vi "Alt_Alpha_Ver 2.0.vi"() -> ()   [LabVIEW 2015]
uses:
  <instrlib>/Keithley 622x LV 2009/Configure/Units/Typedefs/KE622x -- Voltage Meas Units.ctl
  <instrlib>/Keithley 622x LV 2009/Configure/2182 -A/Low Level/Typedefs/KE2182 -- Voltage Ranges.ctl
  <instrlib>/Keithley 622x LV 2009/Configure/2182 -A/Low Level/Typedefs/KE2182 -- Filter Type.ctl
  <instrlib>/Keithley 622x LV 2009/Configure/2182 -A/Low Level/Typedefs/KE2182 -- Filter Count.ctl
  <instrlib>/Keithley 622x LV 2009/Configure/2182 -A/Low Level/Typedefs/KE2182 -- Filter Window.ctl
  <instrlib>/Keithley 622x LV 2009/Configure/2182 -A/Low Level/Typedefs/KE2182 -- NPLCs.ctl
  <instrlib>/Keithley 622x LV 2009/Configure/Units/Typedefs/KE6221 -- PDelta Power Meas Type.ctl
  <instrlib>/Keithley 622x LV 2009/Configure/Delta PDelta DCon Modes/Typedefs/KE6221 -- PDelta Mode Params.ctl
  <instrlib>/Keithley 622x LV 2009/Configure/Delta PDelta DCon Modes/Low Level/Typedefs/KE622x -- Delta PDelta Mode High Level.ctl
  <instrlib>/Keithley 622x LV 2009/Configure/Delta PDelta DCon Modes/Low Level/Typedefs/KE622x -- Delta PDelta Mode Low Level.ctl
  <instrlib>/Keithley 622x LV 2009/Configure/Delta PDelta DCon Modes/Low Level/Typedefs/KE6221 -- PDelta Mode Pulse Width.ctl
  <instrlib>/Keithley 622x LV 2009/Configure/Delta PDelta DCon Modes/Low Level/Typedefs/KE6221 -- PDelta Mode Source Delay.ctl
  <instrlib>/Keithley 622x LV 2009/Configure/Delta PDelta DCon Modes/Low Level/Typedefs/KE622x -- Delta PDelta Mode Num Cycles Mode.ctl
  <instrlib>/Keithley 622x LV 2009/Configure/Delta PDelta DCon Modes/Low Level/Typedefs/KE622x -- Delta PDelta Mode Num Cycles.ctl
  <instrlib>/Keithley 622x LV 2009/Configure/Delta PDelta DCon Modes/Low Level/Typedefs/KE6221 -- PDelta Mode Ranging Mode.ctl
  <instrlib>/Keithley 622x LV 2009/Configure/Delta PDelta DCon Modes/Low Level/Typedefs/KE6221 -- PDelta Mode Num Low Meas.ctl
  <instrlib>/Keithley 622x LV 2009/Configure/Delta PDelta DCon Modes/Low Level/Typedefs/KE6221 -- PDelta Mode Pulse Period.ctl
  <instrlib>/Keithley 622x LV 2009/Configure/Format/Typedefs/KE622x -- Optional Meas Elements.ctl
  <instrlib>/Keithley 622x LV 2009/Configure/Trace Buf/Low Level/Typedefs/KE622x -- Trace Buf.ctl
  <instrlib>/Keithley 622x LV 2009/Configure/Delta PDelta DCon Modes/Typedefs/KE622x -- Delta Mode Params.ctl
  <instrlib>/Keithley 622x LV 2009/Configure/Delta PDelta DCon Modes/Low Level/Typedefs/KE622x -- Delta DCon Mode Delay.ctl
  <instrlib>/Keithley 622x LV 2009/Utility/Typedefs/KE622x -- Instrument Type.ctl
  <instrlib>/Keithley 622x LV 2009/Keithley 622x.lvlib
panel:
  out "FILE":refnum<file>
  out "Reading":sgl[](array[numeric])
  out "Trace Buf":T1 {"Average Voltage (V)" format="%.3p"; "Source Val (A)" format="%.3p"; "Timestamp (secs)" format="%.3f"; "Reading" format="%.7f"}
  in  "Meas Elements To Return":T2={"Timstamp?"=TRUE, "Reading Num?"=TRUE, "Source Value?"=FALSE, "Compliance?"=FALSE, "Average Voltage?"=FALSE}
  in  "stop":bool
  in  "Check For SCPI Errors? (T)":bool=TRUE
  in  "Power Meas Type":T3
  in  "2812 -A Params In":T9={"Auto Range?"=FALSE, "Man / Selected\nRange"=enum."10mV", "Enable Digital\nFilter?"=FALSE, "Filter Type"=enum."Moving", "Filter Count"=10, "Filter\nWindow (%)"=0.01, "Enable Analog\nFilter?"=FALSE, "NPLCs"=5} {"Filter\nWindow (%)" min=0.0 max=10.0 step=0.01 format="%.2f"; "Filter Count" min=1 max=100; "NPLCs" min=1 max=10}
  in  "Measurement Units":T10
  in  "Measurements control":enum32{"PULSE", " DELTA"}(tab)
  in  "Pulsed Delta Mode Params In":T11={"High Level (A)"=0.001, "Low Level (A)"=0.0, "Pulse Width (s)"=0.00011, "Source Delay (s)"=1.6e-05, "Num Cycles Mode"=enum."Infinite", "Finite Count"=1, "Ranging Mode"=enum."Best", "Num Low Meas Per Cycle"=enum."1", "Pulse Period (Num PLCs)"=5, "Pulse Sweep Mode Enabled?"=FALSE} {"Pulse Period (Num PLCs)" min=5 max=999990; "Source Delay (s)" min=1.6e-05 max=0.011966 format="%.3p"; "Pulse Width (s)" min=5e-05 max=0.012 format="%.3p"; "Finite Count" min=2 max=65536; "Low Level (A)" min=-0.105 max=0.0 format="%.3p"; "High Level (A)" min=0.0 max=0.105 format="%.3p"}
  in  "Delta Mode Params In":T21={"High Level (A)"=0.001, "Low Level (A)"=-0.001, "Delay (s)"=0.002, "Num Cycles Mode"=enum."Finite Count", "Finite Count"=1, "Abort On\nCompliance?"=FALSE, "Cold Swithing\nMode Enabled?"=FALSE} {"Finite Count" min=1 max=65536; "Low Level (A)" min=-0.105 max=0.0 format="%.3p"; "High Level (A)" min=0.0 max=0.105 format="%.3p"; "Delay (s)" min=0.001 max=9999.999 format="%.3f"}
  in  "Comments":string
  in  "Folder \nPrename":string
  # "Keithley  6221 & 2182A Measurement System"
  # "FILE CONFIGURATION"
  # "PRE EXPERIMENT CONFIGS"
  # "*** NOTE:  \"Average Voltage\"\nis only available for Differential\nConductance measurements."
  # "*** NOTE:  \"Average Voltage\"\nis only available for Differential\nConductance measurements."
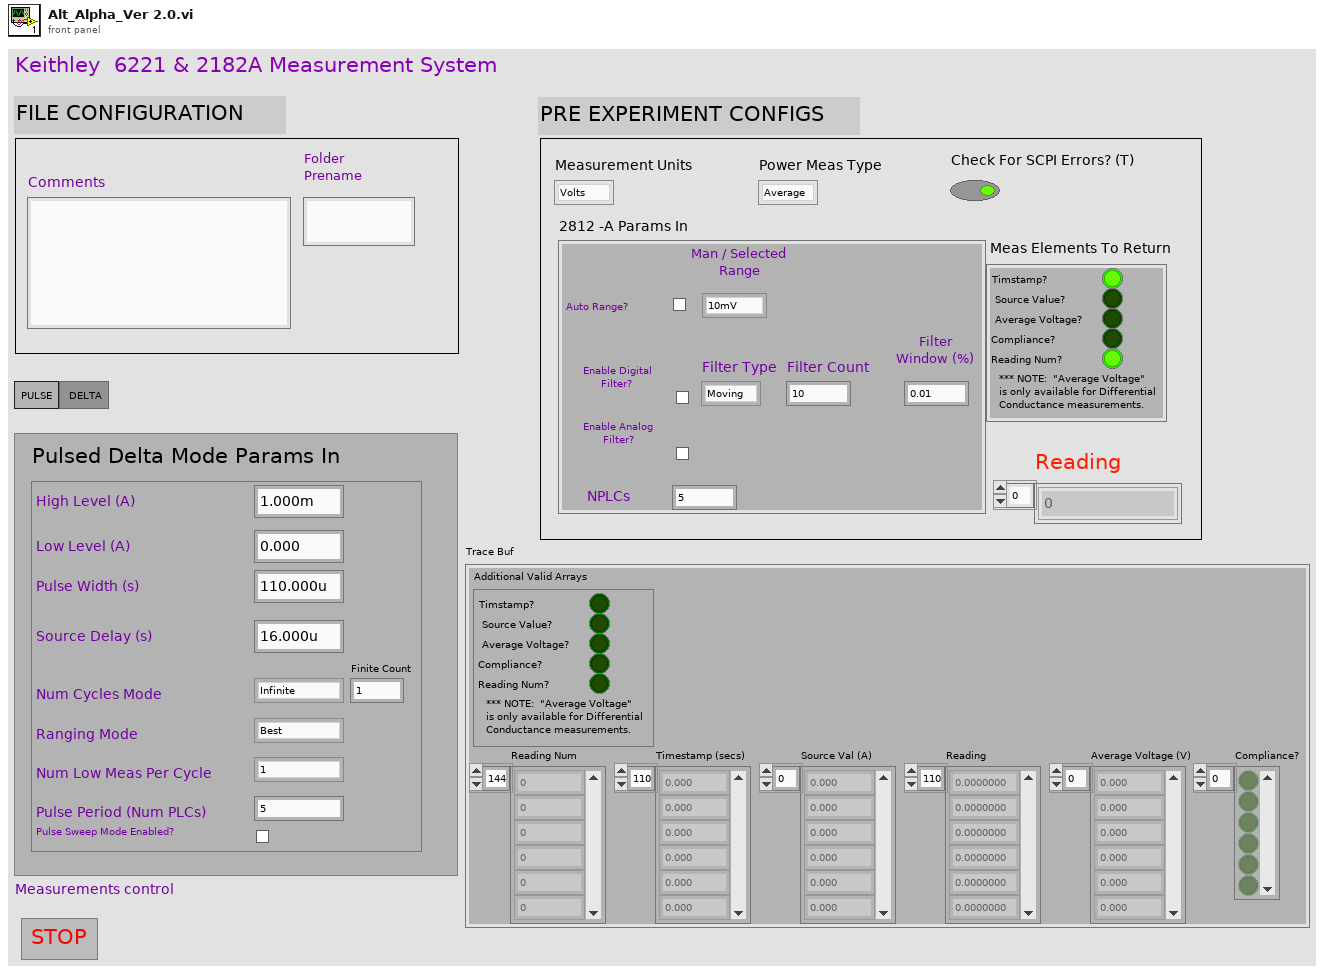
[diagram p1: front panel]
types:
  T1 = typedef "Keithley 622x.lvlib/KE622x -- Trace Buf.ctl" = cluster{"Additional Valid Arrays":T2, "Reading Num":u32[], "Timestamp (secs)":sgl[], "Source Val (A)":sgl[], "Reading":sgl[], "Average Voltage (V)":sgl[], "Compliance?":bool[]}
  T2 = typedef "Keithley 622x.lvlib/KE622x -- Optional Meas Elements.ctl" = cluster{"Timstamp?":bool, "Reading Num?":bool, "Source Value?":bool, "Compliance?":bool, "Average Voltage?":bool}
  T3 = typedef "Keithley 622x.lvlib/KE6221 -- PDelta Power Meas Type.ctl" = enum16{"Average", "Peak"}
  T4 = typedef "Keithley 622x.lvlib/KE2182 -- Voltage Ranges.ctl" = enum16{"10mV", "100mV", "1V", "10V", "100V"}
  T5 = typedef "Keithley 622x.lvlib/KE2182 -- Filter Type.ctl" = enum16{"Moving", "Repeat"}
  T6 = typedef "Keithley 622x.lvlib/KE2182 -- Filter Count.ctl" = u32
  T7 = typedef "Keithley 622x.lvlib/KE2182 -- Filter Window.ctl" = dbl
  T8 = typedef "Keithley 622x.lvlib/KE2182 -- NPLCs.ctl" = u32
  T9 = cluster{"Auto Range?":bool, "Man / Selected\nRange":T4, "Enable Digital\nFilter?":bool, "Filter Type":T5, "Filter Count":T6, "Filter\nWindow (%)":T7, "Enable Analog\nFilter?":bool, "NPLCs":T8}
  T10 = typedef "Keithley 622x.lvlib/KE622x -- Voltage Meas Units.ctl" = enum16{"Volts", "Ohms", "Watts", "Siemens"}
  T11 = typedef "Keithley 622x.lvlib/KE6221 -- PDelta Mode Params.ctl" = cluster{"High Level (A)":T12, "Low Level (A)":T13, "Pulse Width (s)":T14, "Source Delay (s)":T15, "Num Cycles Mode":T16, "Finite Count":T17, "Ranging Mode":T18, "Num Low Meas Per Cycle":T19, "Pulse Period (Num PLCs)":T20, "Pulse Sweep Mode Enabled?":bool}
  T12 = typedef "Keithley 622x.lvlib/KE622x -- Delta PDelta Mode High Level.ctl" = dbl
  T13 = typedef "Keithley 622x.lvlib/KE622x -- Delta PDelta Mode Low Level.ctl" = dbl
  T14 = typedef "Keithley 622x.lvlib/KE6221 -- PDelta Mode Pulse Width.ctl" = dbl
  T15 = typedef "Keithley 622x.lvlib/KE6221 -- PDelta Mode Source Delay.ctl" = dbl
  T16 = typedef "Keithley 622x.lvlib/KE622x -- Delta PDelta Mode Num Cycles Mode.ctl" = enum16{"Finite Count", "Infinite"}
  T17 = typedef "Keithley 622x.lvlib/KE622x -- Delta PDelta Mode Num Cycles.ctl" = u32
  T18 = typedef "Keithley 622x.lvlib/KE6221 -- PDelta Mode Ranging Mode.ctl" = enum16{"Best", "Fixed"}
  T19 = typedef "Keithley 622x.lvlib/KE6221 -- PDelta Mode Num Low Meas.ctl" = enum16{"1", "2"}
  T20 = typedef "Keithley 622x.lvlib/KE6221 -- PDelta Mode Pulse Period.ctl" = u32
  T21 = typedef "Keithley 622x.lvlib/KE622x -- Delta Mode Params.ctl" = cluster{"High Level (A)":T12, "Low Level (A)":T13, "Delay (s)":T22, "Num Cycles Mode":T16, "Finite Count":T17, "Abort On\nCompliance?":bool, "Cold Swithing\nMode Enabled?":bool}
  T22 = typedef "Keithley 622x.lvlib/KE622x -- Delta DCon Mode Delay.ctl" = dbl
  T23 = typedef "Keithley 622x.lvlib/KE622x -- Instrument Type.ctl" = enum16{"KE6220", "KE6221"}
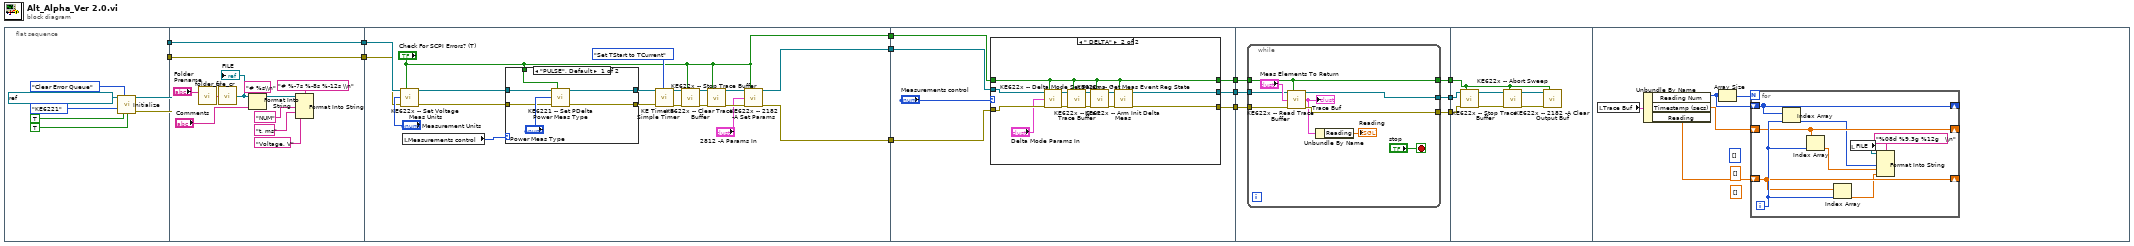
[diagram p0: block diagram]
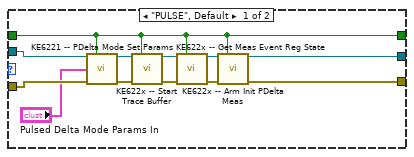
[diagram p3: hidden frame]
diagram:
  n1 = flat-sequence {
    tunnel: [w15] -> w4
    tunnel: [w14] -> w2
    tunnel: w4 -> [w32]
    tunnel: [w32] -> w3
    tunnel: w2 -> [w31]
    tunnel: [w31] -> w1
    tunnel: w3 -> [w50]
    tunnel: w1 -> [w49]
    tunnel: [w40] -> w13
    tunnel: [w39] -> w12
    tunnel: ["Check For SCPI Errors? (T)"] -> w11
    tunnel: w13 -> [w64]
    tunnel: w12 -> [w65]
    tunnel: w11 -> [w63]
    tunnel: [w62] -> w10
    tunnel: [w61] -> w9
    tunnel: [w60] -> w8
    tunnel: w10 -> [w96]
    tunnel: w9 -> [w95]
    tunnel: w8 -> [w94]
    tunnel: [w93] -> w7
    tunnel: [w92] -> w6
    tunnel: [w91] -> w5
    tunnel: w7 -> [w108]
    tunnel: w6 -> [w107]
    tunnel: w5 -> [w106]
    frame #0 {
      n2 = call <instrlib>:"Initialize.vi"("VISA resource name"=refnum<visa-resource-name> "DC_AC_Current_Source_6221", "Error Queue Option"=enum16{"Clear Error Queue", "Error Query"}."Clear Error Queue", "Instrument Type"=KE622x_--_Instrument_Type."KE6221", "ID Query? (T)"=TRUE, "Reset? (T)"=TRUE) -> ("VISA resource name out"=w15:refnum<visa-resource-name>, "error out"=w14:errorcluster)  [unwired: 9 in]
    }
    frame #1 {
      n3 = call "folder_cr.vi"("Name"="Folder \nPrename") -> ("String"=w23:string)
      n4 = call "file_cr.vi"("String"=w23) -> ("refnum out"=w21:refnum<file>)
      "FILE" <- w21
      n5 = Format Into String(format string="# %s\\n", initial string=w21, "Comments") -> (resulting string=w28:refnum<file>)  [unwired: 1 in, 1 out]
      n6 = Format Into String(format string="# %-7s %-8s %-12s \\n", initial string=w28, "NUM" ("input 1"), "t, ms" ("input 2"), "Voltage, V" ("input 3")) -> ()  [unwired: 1 in, 2 out]
    }
    frame #2 {
      n7 = call <instrlib>:"KE622x -- Set Voltage Meas Units.vi"("Resource In"=w50, "Check For SCPI Errors? (T)"="Check For SCPI Errors? (T)", "Voltage Meas Units"="Measurement Units", "error in (no error)"=w49) -> ("Resource Out (dupl)"=w36:refnum<visa-resource-name>, "error out"=w35:errorcluster)  [unwired: 10 in]
      n8 = local read "Measurements control"() -> (w38:enum32{"PULSE", " DELTA"})
      n9 = case shown="\"PULSE\", Default" w38 {
        tunnel: "Check For SCPI Errors? (T)" -> [w56 _]
        tunnel: w36 -> [w55 w59]
        tunnel: w35 -> [w54 w58]
        tunnel: [w53 w59] -> w34
        tunnel: [w52 w58] -> w33
        frame "PULSE", Default {
          n10 = call <instrlib>:"KE6221 -- Set PDelta Power Meas Type.vi"("6221 Resource In"=w55, "Check For SCPI Errors? (T)"=w56, "Power Meas Type"="Power Meas Type", "error in (no error)"=w54) -> ("6221 Resource Out (dupl)"=w53:refnum<visa-resource-name>, "error out"=w52:errorcluster)  [unwired: 10 in]
        }
        frame " DELTA" {
        }
      }
      n11 = call <instrlib>:"KE Timer -- Simple Timer.vi"("Resource In"=w34, "error in (no error)"=w33, "Action"=enum16{"Set TStart to TCurrent", "Get Deltas"}."Set TStart to TCurrent") -> ("Resource Out (dupl)"=w47:refnum<visa-resource-name>, "error out (dupl)"=w46:errorcluster)  [unwired: 7 in, 8 out]
      n12 = call <instrlib>:"KE622x -- Stop Trace Buffer.vi"("Resource In"=w47, "Check For SCPI Errors? (T)"="Check For SCPI Errors? (T)", "error in (no error)"=w46) -> ("Resource Out (dupl)"=w45:refnum<visa-resource-name>, "error out"=w44:errorcluster)  [unwired: 11 in]
      n13 = call <instrlib>:"KE622x -- Clear Trace Buffer.vi"("Resource In"=w45, "Check For SCPI Errors? (T)"="Check For SCPI Errors? (T)", "error in (no error)"=w44) -> ("Resource Out (dupl)"=w43:refnum<visa-resource-name>, "error out"=w42:errorcluster)  [unwired: 11 in]
      n14 = call <instrlib>:"KE622x -- 2182 -A Set Params.vi"("622x Resource In"=w43, "Check For SCPI Errors? (T)"="Check For SCPI Errors? (T)", "2812 -A Params In"="2812 -A Params In", "error in (no error)"=w42) -> ("622x Resource Out (dupl)"=w40:refnum<visa-resource-name>, "error out"=w39:errorcluster)  [unwired: 9 in, 1 out]
    }
    frame #3 {
      n15 = case shown="\" DELTA\"" "Measurements control" {
        tunnel: w65 -> [w77 w81]
        tunnel: w64 -> [w78 w82]
        tunnel: w63 -> [w67 w79]
        tunnel: [w69 w84] -> w62
        tunnel: [w68 w83] -> w61
        tunnel: [w67 w79] -> w60
        frame "PULSE", Default {
          n16 = call <instrlib>:"KE6221 -- PDelta Mode Set Params.vi"("6221 Resource In"=w78, "Check For SCPI Errors? (T)"=w67, "Pulsed Delta Mode Params In"="Pulsed Delta Mode Params In", "error in (no error)"=w77) -> ("6221 Resource Out (dupl)"=w75:refnum<visa-resource-name>, "error out"=w74:errorcluster)  [unwired: 9 in, 1 out]
          n17 = call <instrlib>:"KE622x -- Start Trace Buffer.vi"("Resource In"=w75, "Check For SCPI Errors? (T)"=w67, "error in (no error)"=w74) -> ("Resource Out (dupl)"=w73:refnum<visa-resource-name>, "error out"=w72:errorcluster)  [unwired: 11 in]
          n18 = call <instrlib>:"KE622x -- Get Meas Event Reg State.vi"("VISA Resource In"=w73, "Error Query (T)?"=w67, "error in (no error)"=w72) -> ("VISA Resource Out (dupl)"=w71:refnum<visa-resource-name>, "error out"=w70:errorcluster)  [unwired: 10 in, 1 out]
          n19 = call <instrlib>:"KE622x -- Arm Init PDelta Meas.vi"("Resource In"=w71, "Check For SCPI Errors? (T)"=w67, "error in (no error)"=w70) -> ("Resource Out (dupl)"=w69:refnum<visa-resource-name>, "error out"=w68:errorcluster)  [unwired: 11 in]
        }
        frame " DELTA" {
          n20 = call <instrlib>:"KE622x -- Delta Mode Set Params.vi"("Resource In"=w82, "Check For SCPI Errors? (T)"=w79, "Delta Mode Params In"="Delta Mode Params In", "error in (no error)"=w81) -> ("Resource Out (dupl)"=w85:refnum<visa-resource-name>, "error out"=w88:errorcluster)  [unwired: 9 in, 1 out]
          n21 = call <instrlib>:"KE622x -- Start Trace Buffer.vi"("Resource In"=w85, "Check For SCPI Errors? (T)"=w79, "error in (no error)"=w88) -> ("Resource Out (dupl)"=w86:refnum<visa-resource-name>, "error out"=w89:errorcluster)  [unwired: 11 in]
          n22 = call <instrlib>:"KE622x -- Get Meas Event Reg State.vi"("VISA Resource In"=w86, "Error Query (T)?"=w79, "error in (no error)"=w89) -> ("VISA Resource Out (dupl)"=w87:refnum<visa-resource-name>, "error out"=w90:errorcluster)  [unwired: 10 in, 1 out]
          n23 = call <instrlib>:"KE622x -- Arm Init Delta Meas.vi"("Resource In"=w87, "Check For SCPI Errors? (T)"=w79, "error in (no error)"=w90) -> ("Resource Out (dupl)"=w84:refnum<visa-resource-name>, "error out"=w83:errorcluster)  [unwired: 11 in]
        }
      }
    }
    frame #4 {
      n24 = while {
        tunnel: w96 -> [w102]
        tunnel: w95 -> [w103]
        tunnel: w94 -> [w101]
        tunnel: [w101] -> w93
        tunnel: [w100] -> w92
        tunnel: [w99] -> w91
        stop <- "stop" stop-if-true
        n25 = call <instrlib>:"KE622x -- Read Trace Buffer.vi"("Resource In"=w102, "Check For SCPI Errors? (T)"=w101, "Meas Elements To Return"="Meas Elements To Return", "error in (no error)"=w103) -> ("Resource Out (dupl)"=w100:refnum<visa-resource-name>, "Trace Buf"=w98:T1, "error out"=w99:errorcluster)  [unwired: 9 in]
        "Trace Buf" <- w98
        n26 = Unbundle By Name(w98) -> ("Reading"=→"Reading":sgl[])
      }
    }
    frame #5 {
      n27 = call <instrlib>:"KE622x -- Stop Trace Buffer.vi"("Resource In"=w107, "Check For SCPI Errors? (T)"=w108, "error in (no error)"=w106) -> ("Resource Out (dupl)"=w112:refnum<visa-resource-name>, "error out"=w110:errorcluster)  [unwired: 11 in]
      n28 = call <instrlib>:"KE622x -- Abort Sweep.vi"("Resource In"=w112, "Check For SCPI Errors? (T)"=w108, "error in (no error)"=w110) -> ("Resource Out (dupl)"=w111:refnum<visa-resource-name>, "error out"=w109:errorcluster)  [unwired: 11 in]
      n29 = call <instrlib>:"KE622x -- 2182 -A Clear Output Buf.vi"("622x Resource In"=w111, "Check For SCPI Errors? (T)"=w108, "error in (no error)"=w109) -> ()  [unwired: 10 in, 3 out]
    }
    frame #6 {
      (unwired) dbl[] []
      (unwired) dbl[] []
      (unwired) i32[] []
      n30 = local read "Trace Buf"() -> (w117:T1)
      n31 = Unbundle By Name(w117) -> ("Reading Num"=w113:u32[], "Timestamp (secs)"=w115:sgl[], "Reading"=w114:sgl[])
      n32 = Array Size(array=w113) -> (size(s)=w116:i32)
      n33 = for {
        N: w116 -> [_]
        shift-right: [w125] -> _
        shift-left: w113 -> [w125]
        shift-right: [w124] -> _
        shift-left: w115 -> [w124]
        shift-right: [w123] -> _
        shift-left: w114 -> [w123]
        i -> [w126]
        n34 = Index Array(array=w125, index=w126) -> (element=w120:u32)
        n35 = Index Array(array=w124, index=w126) -> (element=w119:sgl)
        n36 = Index Array(array=w123, index=w126) -> (element=w118:sgl)
        n37 = local read "FILE"() -> (w122:refnum<file>)
        n38 = Format Into String(format string="%08d %9.3g %12g   \\n", initial string=w122, w120, w119, w118) -> ()  [unwired: 1 in, 2 out]
      }
    }
  }
